vi "AuMT8852B Modulation Index Extended Results Query.vi"(7 "Stage":T1(ring), 8 "error in (no error)":errorcluster, 11 "VISA session":refnum<visa-resource-name>) -> (0 "error out":errorcluster, 2 "error code":i32, 3 "VISA session out":refnum<visa-resource-name>, 4 "Results":T2 {"Delta f2 avg / delta f1 avg" format="%.2f"; "Delta f2 average (kHz)" format="%.2f"; "Delta f2 maximum (kHz)" format="%.2f"; "Delta f1 average (kHz)" format="%.2f"; "Delta f1 maximum (kHz)" format="%.2f"})   [LabVIEW 2017]
doc: "Anritsu MT8852B Bluetooth Tester\n\nReturns the results of the Modulation Characteristics test.\n\nINPUTS\nStage - results of the individual hopping stages of the test.\n\nOUTPUTS\nResults - measurements made during the test."
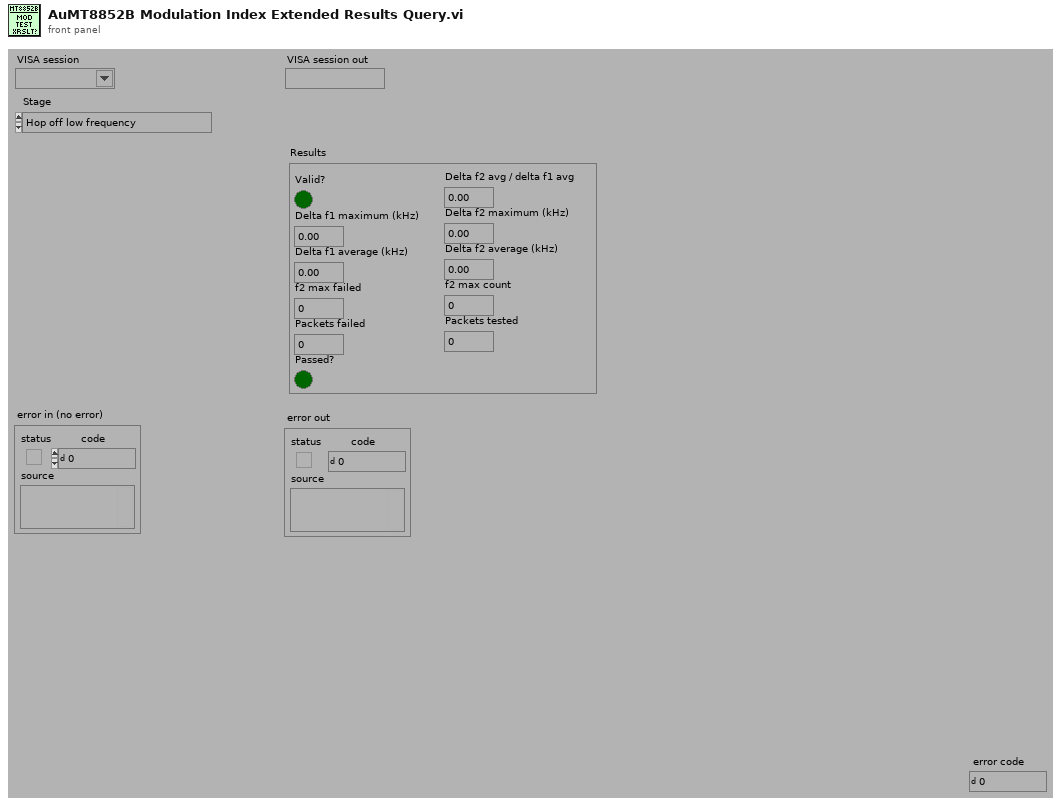
[diagram p1: front panel]
types:
  T1 = enum16{"Hop off low frequency", "Hop off medium frequency", "Hop off high frequency"}
  T2 = cluster{"Delta f1 maximum (kHz)":dbl, "Delta f1 average (kHz)":dbl, "Delta f2 maximum (kHz)":dbl, "Delta f2 average (kHz)":dbl, "Passed?":bool, "Delta f2 avg / delta f1 avg":dbl, "Valid?":bool, "f2 max failed":i32, "f2 max count":i32, "Packets failed":i32, "Packets tested":i32}
  T3 = enum16{"Simulate", "Range check", "Cache", "Query instrument status"}
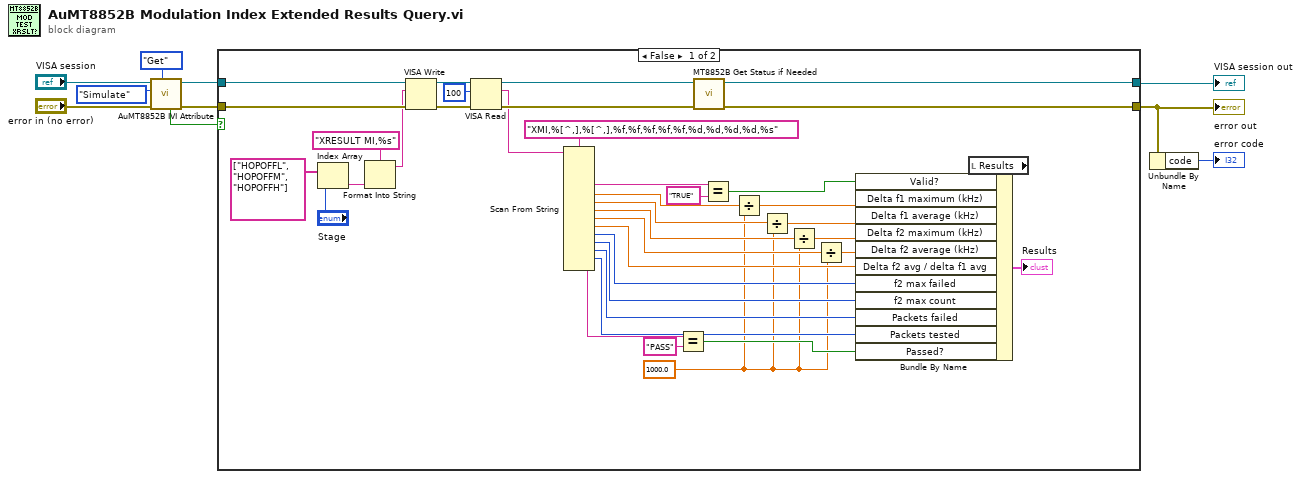
[diagram p0: block diagram]
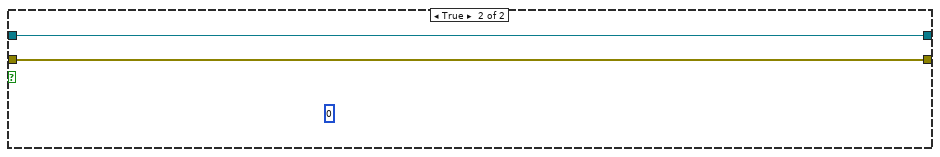
[diagram p2: hidden frame]
diagram:
  n1 = call <instrlib>:"AuMT8852B IVI Attribute.vi"("Set/Get (Set)"=enum16{"Set", "Get"}."Get", "error in (no error)"="error in (no error)", "Flag (Simulate)"=T3."Simulate", "VISA session"="VISA session") -> ("error out"=w7:errorcluster, "VISA session out"=w9:refnum<visa-resource-name>, "Value out"=w3:bool)  [unwired: 5 in]
  n2 = case shown="False" w3 {
    tunnel: [w37 w50] -> w10
    tunnel: [w36 w49] -> w1
    tunnel: w9 -> [w48 w50]
    tunnel: w7 -> [w47 w49]
    frame False {
      w11 = 1000.0 ("y")
      n3 = Index Array(array=string[] ["HOPOFFL", "HOPOFFM", "HOPOFFH"], index="Stage") -> (element=w31:string)
      n4 = Format Into String(format string="XRESULT MI,%s" ("write buffer (\"\")"), w31) -> (resulting string=w22:string)  [unwired: 2 in, 1 out]
      n5 = VISA Write(VISA resource name=w48, write buffer=w22, error in (no error)=w47) -> (VISA resource name out=w46:refnum<visa-resource-name>, error out=w45:errorcluster)  [unwired: 1 out]
      n6 = VISA Read(VISA resource name=w46, byte count=u32 100 ("byte count (0)"), error in (no error)=w45) -> (VISA resource name out=w34:refnum<visa-resource-name>, read buffer=w21:string, error out=w33:errorcluster)  [unwired: 1 out]
      n7 = Scan From String(format string="XMI,%[^,],%[^,],%f,%f,%f,%f,%f,%d,%d,%d,%d,%s" ("Format String"), input string=w21) -> (output 2=w28:string, output 3=w16:dbl, output 4=w15:dbl, output 5=w14:dbl, output 6=w13:dbl, output 7=w12:dbl, output 8=w27:i32, output 9=w26:i32, output 10=w25:i32, output 11=w24:i32, output 12=w23:string)  [unwired: 15 in, 3 out]
      n8 = Equal?(x=w23, y="PASS") -> (x = y?=w35:bool)
      n9 = call <instrlib>:"MT8852B Get Status if Needed.vi"("error in (no error)"=w33, "VISA session"=w34) -> ("error out"=w36:errorcluster, "VISA session out"=w37:refnum<visa-resource-name>)  [unwired: 8 in]
      n10 = Equal?(x=w28, y="TRUE") -> (x = y?=w41:bool)
      n11 = Divide(x=w16, y=w11) -> (x/y=w17:dbl)
      n12 = Divide(x=w15, y=w11) -> (x/y=w18:dbl)
      n13 = Divide(x=w14, y=w11) -> (x/y=w19:dbl)
      n14 = Divide(x=w13, y=w11) -> (x/y=w20:dbl)
      n15 = local read "Results"() -> (w42:T2)
      n16 = Bundle By Name(cluster=w42, "Valid?"=w41, "Delta f1 maximum (kHz)"=w17, "Delta f1 average (kHz)"=w18, "Delta f2 maximum (kHz)"=w19, "Delta f2 average (kHz)"=w20, "Delta f2 avg / delta f1 avg"=w12, "f2 max failed"=w27, "f2 max count"=w26, "Packets failed"=w25, "Packets tested"=w24, "Passed?"=w35) -> (→"Results":T2)
    }
    frame True {
      (unwired) u8 0
    }
  }
  "error out" <- w1
  "VISA session out" <- w10
  n17 = Unbundle By Name(w1) -> ("code"=→"error code":i32)
